vi "Test 2.vi"() -> ()   [LabVIEW 2016]
panel:
  in  "自定义多列表框":T1(xcontrol)
  out "数组":string[][](array[string])
  in  "停止按钮":bool
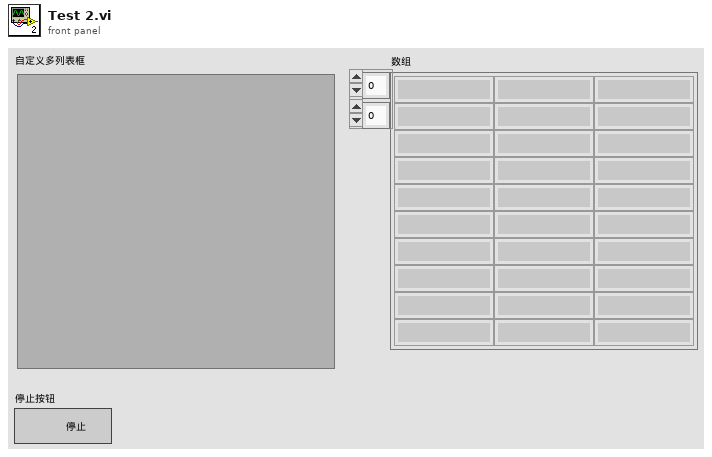
[diagram p1: front panel]
types:
  T1 = cluster{"行首":string[], "列首":string[], "项名":string[][]}
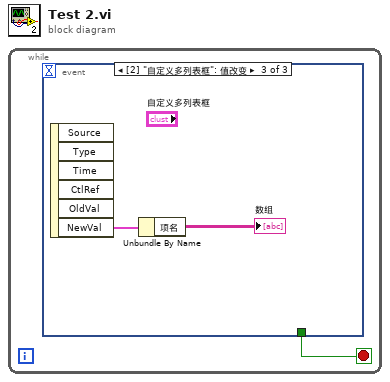
[diagram p0: block diagram]
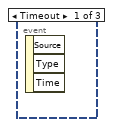
[diagram p2: hidden frame]
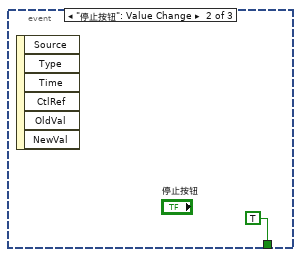
[diagram p3: hidden frame]
diagram:
  n1 = while {
    stop <- w1 stop-if-true
    n2 = event shown="[2] \"自定义多列表框\": 值改变" {
      selector: _ -> [_ _ _]
      dyn-events: _ -> [_ _ _]
      timeout: _ -> [_ _ _]
      tunnel: [_ TRUE _] -> w1
      event Timeout {
        n3 = event-data() -> ()  [unwired: 1 in, 3 out]
      }
      event "停止按钮": Value Change {
        n4 = event-data() -> ()  [unwired: 1 in, 6 out]
      }
      event "自定义多列表框": Value Change {
        n5 = event-data() -> ("NewVal"=w4:T1)  [unwired: 1 in, 5 out]
        n6 = Unbundle By Name(w4) -> ("项名"=→"数组":string[][])
      }
    }
  }
